vi "BaseProvider_IniFileSettings.vi"(1 "IniFileSettings":T1, 5 "error in (no error)":errorcluster, 6 "Action":enum16{"Read", "Load", "Save"}(ring)) -> (15 "IniFileSettings":T1, 19 "error out":errorcluster)   [LabVIEW 2020]
uses:
  <resource>/Framework/Providers/Open_GDS/ClassProviders/Provider_BaseClassInterface/BaseProvider_SubVIs/BaseProvider_IniFileSettings.ctl
  <resource>/Framework/Providers/Open_GDS/ClassProviders/Provider_BaseClassInterface/BaseProvider_SubVIs/BaseProvider_FileNamingOption.ctl
  <vilib>/Utility/config.llb/Read Key (String).vi
  <vilib>/Utility/config.llb/Write Key (String).vi
  <vilib>/Utility/config.llb/NI_LVConfig.lvlib
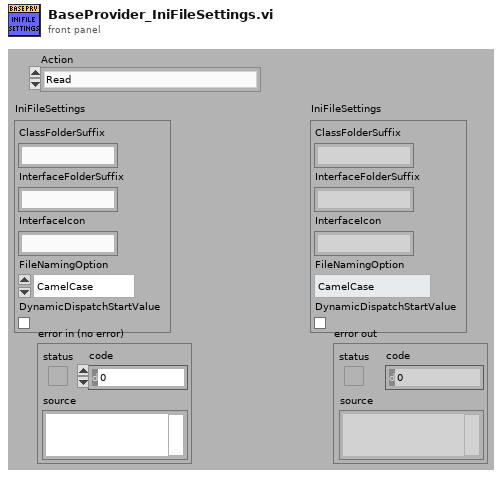
[diagram p1: front panel]
types:
  T1 = typedef "BaseProvider_IniFileSettings.ctl" = cluster{"ClassFolderSuffix":string, "InterfaceFolderSuffix":string, "InterfaceIcon":string, "FileNamingOption":T2, "DynamicDispatchStartValue":bool}
  T2 = typedef "BaseProvider_FileNamingOption.ctl" = enum16{"CamelCase", "Space", "Underscore"}
  T3 = typedef "NI_LVConfig.lvlib/Config Data RefNum.ctl" = refnum<k1>
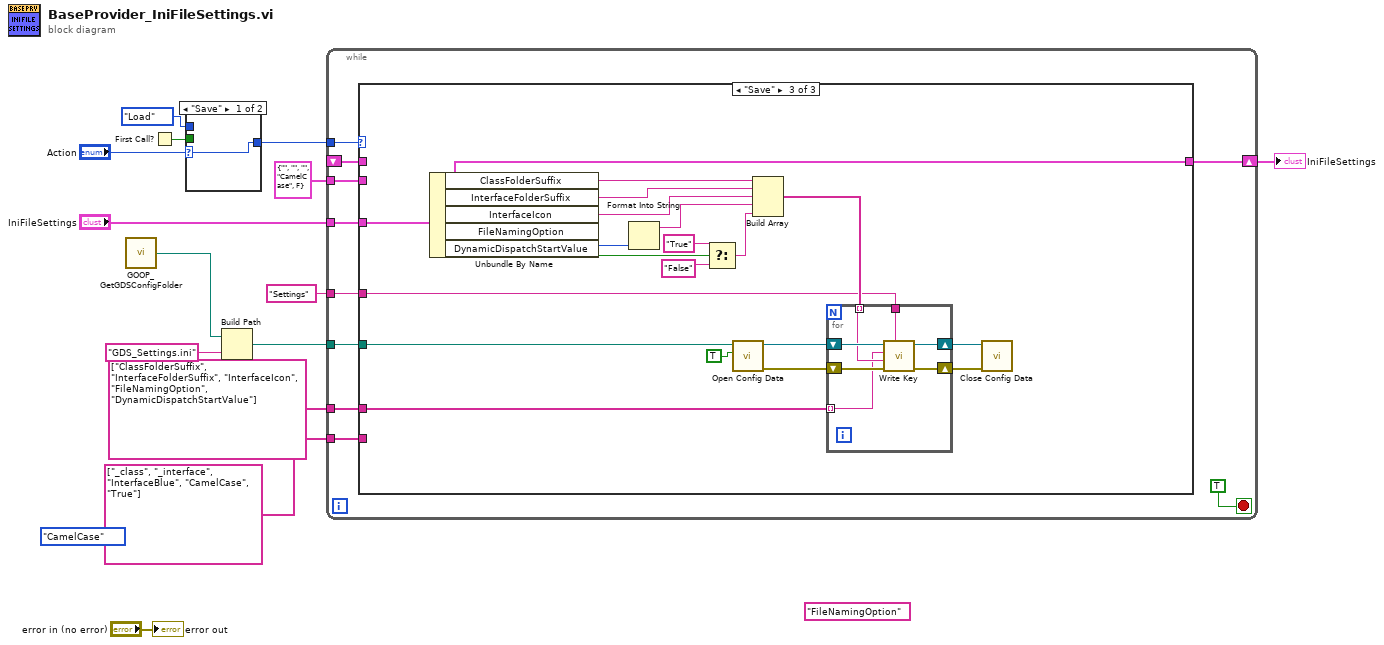
[diagram p0: block diagram]
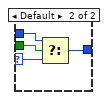
[diagram p2: hidden frame]
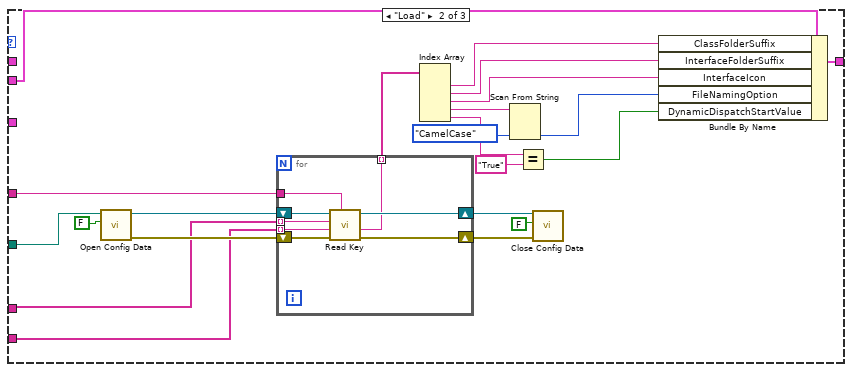
[diagram p4: hidden frame]
diagram:
  (unwired) BaseProvider_FileNamingOption."CamelCase" ("input 1")
  (unwired) "FileNamingOption" ("key")
  n1 = call <resource>:"GOOP_GetGDSConfigFolder.vi"() -> ("GDSFolderPath"=w13:path)
  n2 = First Call?() -> (First Call?: T/F=w10:bool)
  n3 = case shown="\"Save\"" "Action" {
    selector: "Action" -> [w15 w16]
    tunnel: w10 -> [_ w19]
    tunnel: [w15 w18] -> w9
    tunnel: enum16{"Read", "Load", "Save"}."Load" ("t") -> [_ w17]
    frame "Save" {
    }
    frame Default {
      n4 = Select(t=w17, s=w19, f=w16) -> (s? t:f=w18:enum16{"Read", "Load", "Save"})
    }
  }
  n5 = Build Path(base path=w13, name or relative path="GDS_Settings.ini") -> (appended path=w12:path)
  n6 = while {
    tunnel: w9 -> [w29]
    tunnel: w12 -> [w28]
    shift-right: [w26] -> w11
    shift-left: _ -> [w25]
    tunnel: "IniFileSettings" -> [w24]
    tunnel: T1 {"ClassFolderSuffix"="", "InterfaceFolderSuffix"="", "InterfaceIcon"="", "FileNamingOption"=enum."CamelCase", "DynamicDispatchStartValue"=FALSE} ("IniFileSettings") -> [w23]
    tunnel: string[] ["ClassFolderSuffix", "InterfaceFolderSuffix", "InterfaceIcon", "FileNamingOption", "DynamicDispatchStartValue"] -> [w22]
    tunnel: "Settings" ("section") -> [w21]
    tunnel: string[] ["_class", "_interface", "InterfaceBlue", "CamelCase", "True"] -> [w20]
    stop <- TRUE stop-if-true
    n7 = case shown="\"Save\"" w29 {
      tunnel: w28 -> [_ w52 w78]
      tunnel: [w30 w47 w66] -> w26
      tunnel: w25 -> [w30 _ _]
      tunnel: w24 -> [_ _ w66]
      tunnel: w23 -> [_ w48 _]
      tunnel: w22 -> [_ w44 w67]
      tunnel: w21 -> [_ w45 w65]
      tunnel: w20 -> [_ w43 _]
      frame "Read", Default {
      }
      frame "Load" {
        n8 = call <vilib>:"Open Config Data.vi"("create file if necessary (T)"=FALSE, "configuration file path"=w52) -> ("error out"=w50:errorcluster, "refnum"=w51:T3)  [unwired: 7 in, 1 out]
        n9 = for {
          tunnel: w45 -> [w58]
          tunnel: w44 -> [w57] mode=indexing
          tunnel: w43 -> [w56] mode=indexing
          shift-right: [w55] -> w42
          shift-left: w51 -> [w60]
          shift-right: [w54] -> w41
          shift-left: w50 -> [w59]
          tunnel: [w53] -> w40 mode=indexing
          n10 = call-poly <vilib>:"Read Key.vi"("section"=w58, "error in (no error)"=w59, "default value"=w56, "key"=w57, "refnum"=w60) -> ("error out"=w54:errorcluster, "value"=w53:string, "refnum out"=w55:T3)  [unwired: 3 in, 1 out]
        }
        n11 = Index Array(array=w40) -> (element #1=w34:string, element #2=w35:string, element #3=w36:string, element #4=w39:string, element #5=w33:string)  [unwired: 5 in]
        n12 = Scan From String(input string=w39, default 1=BaseProvider_FileNamingOption."CamelCase" ("input 1")) -> (output 1=w37:T2)  [unwired: 3 in, 3 out]
        n13 = Equal?(x=w33, y="True") -> (x = y?=w31:bool)
        n14 = call <vilib>:"Close Config Data.vi"("error in (no error)"=w41, "write file if changed (T)"=FALSE, "refnum"=w42) -> ()  [unwired: 7 in, 2 out]
        n15 = Bundle By Name(cluster=w48, "ClassFolderSuffix"=w34, "InterfaceFolderSuffix"=w35, "InterfaceIcon"=w36, "FileNamingOption"=w37, "DynamicDispatchStartValue"=w31) -> (w47:T1)
      }
      frame "Save" {
        n16 = Unbundle By Name(w66) -> ("ClassFolderSuffix"=w77:string, "InterfaceFolderSuffix"=w76:string, "InterfaceIcon"=w75:string, "FileNamingOption"=w73:T2, "DynamicDispatchStartValue"=w64:bool)
        n17 = Format Into String(w73) -> (resulting string=w74:string)  [unwired: 3 in, 1 out]
        n18 = Select(t="True" ("y"), s=w64, f="False" ("y")) -> (s? t:f=w63:string)
        n19 = call <vilib>:"Open Config Data.vi"("create file if necessary (T)"=TRUE, "configuration file path"=w78) -> ("error out"=w70:errorcluster, "refnum"=w72:T3)  [unwired: 7 in, 1 out]
        n20 = Build Array(w77, w76, w75, w74, w63) -> (w68:string[])
        n21 = for {
          tunnel: w68 -> [w82] mode=indexing
          shift-right: [w85] -> w71
          shift-left: w72 -> [w86]
          shift-right: [w83] -> w69
          shift-left: w70 -> [w84]
          tunnel: w67 -> [w81] mode=indexing
          tunnel: w65 -> [w80]
          n22 = call-poly <vilib>:"Write Key.vi"("section"=w80, "error in (no error)"=w84, "value"=w82, "key"=w81, "refnum"=w86) -> ("error out"=w83:errorcluster, "refnum out"=w85:T3)  [unwired: 4 in, 1 out]
        }
        n23 = call <vilib>:"Close Config Data.vi"("error in (no error)"=w69, "refnum"=w71) -> ()  [unwired: 8 in, 2 out]
      }
    }
  }
  "IniFileSettings" <- w11
  "error out" <- "error in (no error)"
